vi "FTW-Test-JSON-ObjectDelete.vi"() -> (0 "Test Result":errorcluster)   [LabVIEW 2014]
uses:
  src/error/FTW-ERR-Assert-DeveloperError.vi
panel:
  out "Original JSON":string
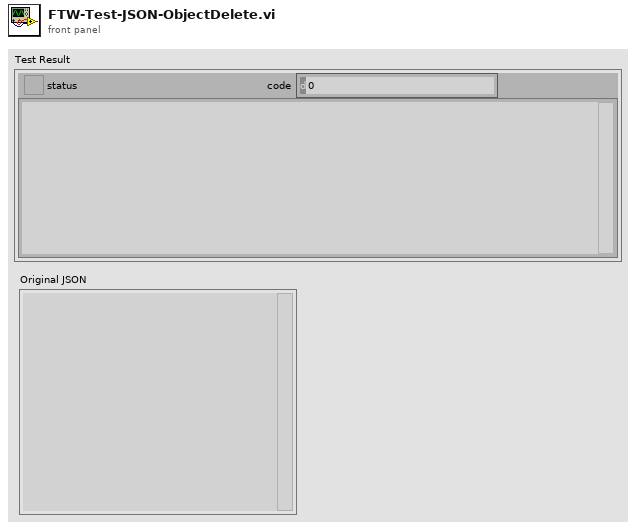
[diagram p1: front panel]
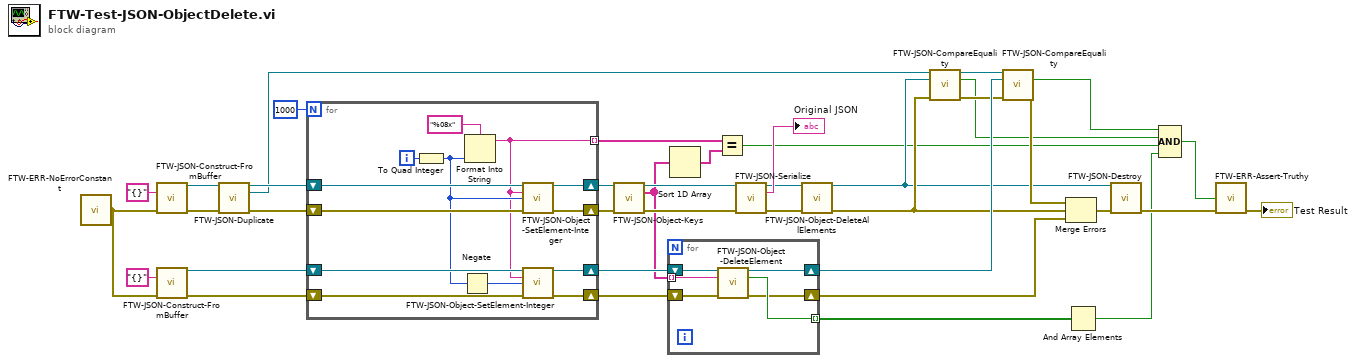
[diagram p0: block diagram]
diagram:
  n1 = call "FTW-ERR-NoErrorConstant.vi"() -> ("no error"=w34:errorcluster)
  n2 = call "FTW-JSON-Construct-FromBuffer.vi"("JSON String (UTF-8)"="{}", "error in"=w34) -> ("JSON Object"=w30:refnum<data-value>, "error out"=w29:errorcluster)  [unwired: 12 in]
  n3 = call "FTW-JSON-Construct-FromBuffer.vi"("JSON String (UTF-8)"="{}", "error in"=w34) -> ("JSON Object"=w32:refnum<data-value>, "error out"=w33:errorcluster)  [unwired: 12 in]
  n4 = call "FTW-JSON-Duplicate.vi"("JSON Object"=w30, "error in"=w29) -> ("JSON Object out"=w27:refnum<data-value>, "Duplicated JSON Object"=w15:refnum<data-value>, "error out"=w28:errorcluster)  [unwired: 11 in]
  n5 = for {
    N: 1000 -> [_]
    shift-right: [w49] -> w24
    shift-left: w28 -> [w50]
    shift-right: [w51] -> w26
    shift-left: w27 -> [w52]
    shift-right: [w44] -> w19
    shift-left: w33 -> [w46]
    shift-right: [w45] -> w20
    shift-left: w32 -> [w47]
    tunnel: [w40] -> w21 mode=indexing
    i -> [w48]
    n6 = To Quad Integer(1:w48) -> (0:w41:i64)
    n7 = Negate(x=w41) -> (-x=w42:i64)
    n8 = Format Into String(format string="%08x", w41) -> (resulting string=w40:string)  [unwired: 2 in, 1 out]
    n9 = call "FTW-JSON-Object-SetElement-Integer.vi"("JSON Object"=w52, "Key"=w40, "Value"=w41, "error in"=w50) -> ("JSON Object out"=w51:refnum<data-value>, "error out"=w49:errorcluster)  [unwired: 10 in]
    n10 = call "FTW-JSON-Object-SetElement-Integer.vi"("JSON Object"=w47, "Key"=w40, "Value"=w42, "error in"=w46) -> ("JSON Object out"=w45:refnum<data-value>, "error out"=w44:errorcluster)  [unwired: 10 in]
  }
  n11 = call "FTW-JSON-Object-Keys.vi"("JSON Object"=w26, "error in"=w24) -> ("JSON Object out"=w25:refnum<data-value>, "Keys"=w18:string[], "error out"=w23:errorcluster)  [unwired: 11 in]
  n12 = for {
    shift-right: [w54] -> w13
    shift-left: w20 -> [w58]
    shift-right: [w53] -> w9
    shift-left: w19 -> [w57]
    tunnel: [w56] -> w1 mode=indexing
    tunnel: w18 -> [w55] mode=indexing
    n13 = call "FTW-JSON-Object-DeleteElement.vi"("JSON Object"=w58, "Key"=w55, "error in"=w57) -> ("JSON Object out"=w54:refnum<data-value>, "Found and Removed?"=w56:bool, "error out"=w53:errorcluster)  [unwired: 10 in]
  }
  n14 = Sort 1D Array(array=w18) -> (sorted array=w22:string[])
  n15 = Equal?(x=w21, y=w22) -> (x = y?=w4:bool)
  n16 = call "FTW-JSON-Serialize.vi"("JSON Object"=w25, "error in"=w23) -> ("JSON Object out"=w17:refnum<data-value>, "JSON String (UTF-8)"=→"Original JSON":string, "error out"=w16:errorcluster)  [unwired: 11 in]
  n17 = call "FTW-JSON-Object-DeleteAllElements.vi"("JSON Object"=w17, "error in"=w16) -> ("JSON Object out"=w7:refnum<data-value>, "error out"=w10:errorcluster)  [unwired: 12 in]
  n18 = call "FTW-JSON-CompareEquality.vi"("JSON Object"=w15, "JSON Object to Compare"=w7, "error in"=w10) -> ("JSON Object out"=w14:refnum<data-value>, "Equal?"=w5:bool, "error out"=w12:errorcluster)  [unwired: 10 in]
  n19 = call "FTW-JSON-CompareEquality.vi"("JSON Object"=w14, "JSON Object to Compare"=w13, "error in"=w12) -> ("Equal?"=w6:bool, "error out"=w11:errorcluster)  [unwired: 10 in, 1 out]
  n20 = Merge Errors(w11, w10, w9) -> (w8:errorcluster)
  n21 = And Array Elements(Boolean array=w1) -> (logical AND=w2:bool)
  n22 = call "FTW-JSON-Destroy.vi"("JSON Object"=w7, "error in"=w8) -> ("error out"=w31:errorcluster)  [unwired: 13 in]
  n23 = Compound Arithmetic op=AND(w6, w5, w4, w2) -> (w3:bool)
  n24 = call "FTW-ERR-Assert-Truthy.vi"("Expected Truthy"=w3, "error in"=w31) -> ("error out"=→"Test Result":errorcluster)  [unwired: 13 in]
